vi "OpenGetAttirbutes.vi"   [LabVIEW 2020]
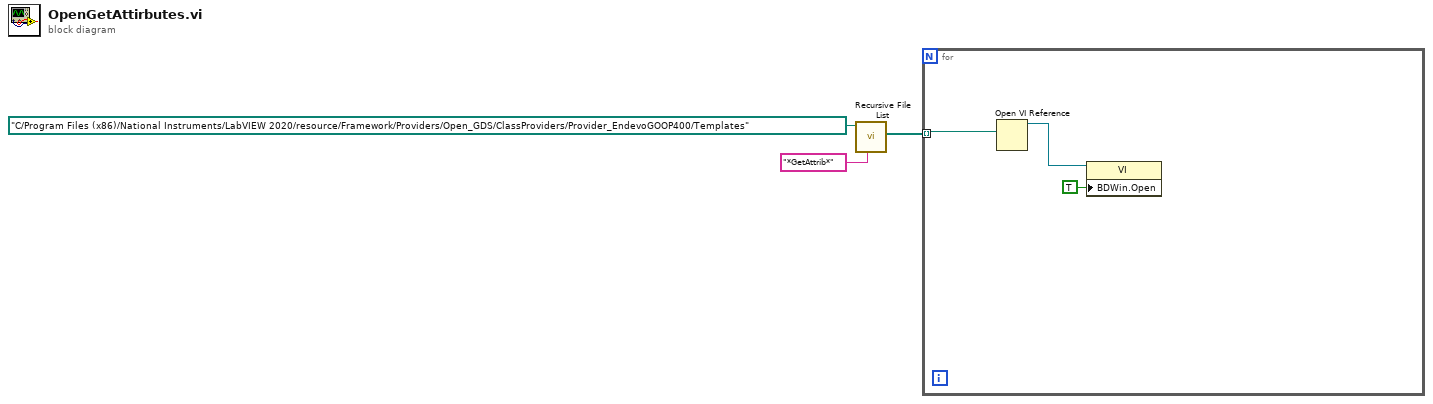
[diagram p0: block diagram]
diagram:
  n1 = call <vilib>:"Recursive File List.vi"("pattern"="*GetAttrib*", "Folder Path"=path "C:/Program Files (x86)/National Instruments/LabVIEW 2020/resource/Framework/Providers/Open_GDS/ClassProviders/Provider_EndevoGOOP400/Templates") -> ("All Files in Dir"=w1:path[])  [unwired: 5 in, 4 out]
  n2 = for {
    tunnel: w1 -> [w6] mode=indexing
    n3 = Open VI Reference(vi path=w6) -> (vi reference=w5:refnum<vi>)  [unwired: 5 in, 1 out]
    n4 = property class="VI"(reference=w5, "BDWin.Open"=TRUE ("Block Diagram Window:Open")) -> ()  [unwired: 1 in, 2 out]
  }
